vi "Choreo_TrajectorySwerve_Equals.vi"(9 "otherChoreoTrajectorySwerve":T1, 11 "ChoreoTrajectorySwerve":T1) -> (3 "equal":bool)   [LabVIEW 2019, in "ChoreoLib.lvlib"]
doc: "Return total time duration of this trajectory\n\nInputs: \n - ChoreoTrajectory - cluster - Input trajectory\n\nOutputs:\n - TotalTime - double - The total time duration of this trajectory.\n."
uses:
  TypeDef/ChoreoTrajectorySwerve.ctl
  TypeDef/ChoreoSwerveSample.ctl
  TypeDef/ChoreoEventMarker.ctl
  ChoreoLib.lvlib
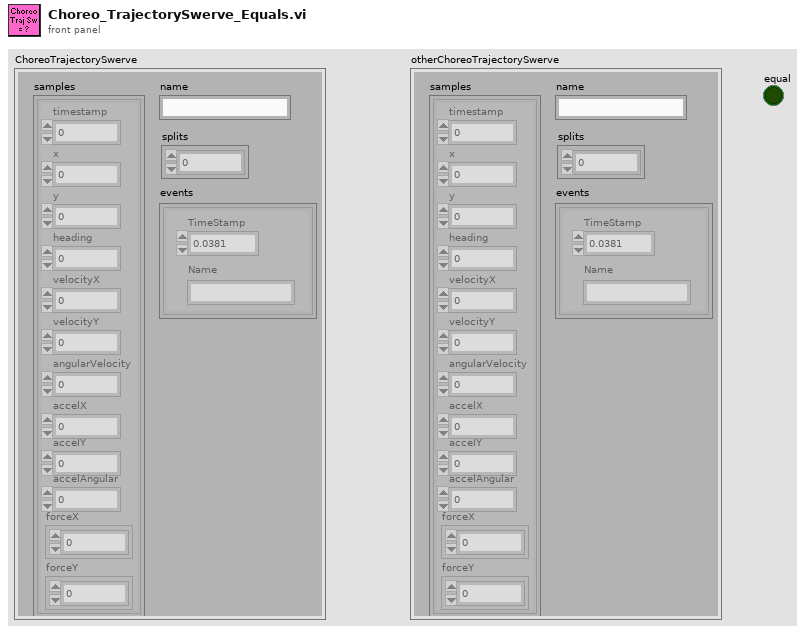
[diagram p1: front panel]
types:
  T1 = typedef "ChoreoLib.lvlib/ChoreoTrajectorySwerve.ctl" = cluster{"name":string, "samples":T2[], "splits":i32[], "events":T3[]}
  T2 = typedef "ChoreoLib.lvlib/ChoreoSwerveSample.ctl" = cluster{"timestamp":dbl, "x":dbl, "y":dbl, "heading":dbl, "velocityX":dbl, "velocityY":dbl, "angularVelocity":dbl, "accelX":dbl, "accelY":dbl, "accelAngular":dbl, "forceX":dbl[], "forceY":dbl[]}
  T3 = typedef "ChoreoLib.lvlib/ChoreoEventMarker.ctl" = cluster{"TimeStamp":dbl, "Name":string}
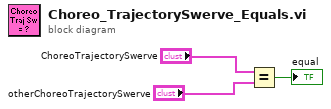
[diagram p0: block diagram]
diagram:
  n1 = Equal?(x="ChoreoTrajectorySwerve", y="otherChoreoTrajectorySwerve") -> (x = y?=→"equal":bool)
